vi "LINC Error.vi"(8 "error in (no error)":errorcluster, 10 "expanded error (F)":bool, 11 "LINC session":refnum<class "LINC.lvclass">) -> (0 "error out":errorcluster, 3 "dup LINC session":refnum<class "LINC.lvclass">)   [LabVIEW 2018, in "STEPkgDriver_LINC.lvlib" / "LINC.lvclass"]
uses:
  LINC.lvclass
  STEPkgDriver_LINC.lvlib
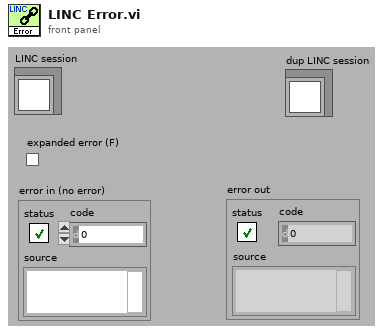
[diagram p1: front panel]
types:
  T1 = cluster{"binary value (F)":bool, "include unit (F)":bool}
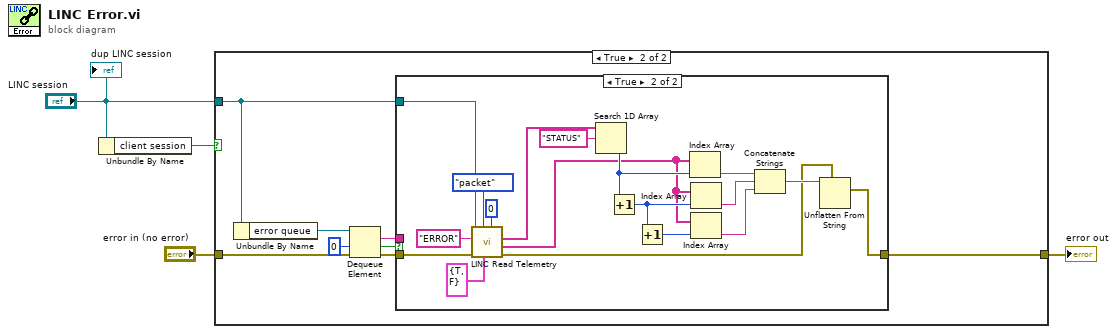
[diagram p0: block diagram]
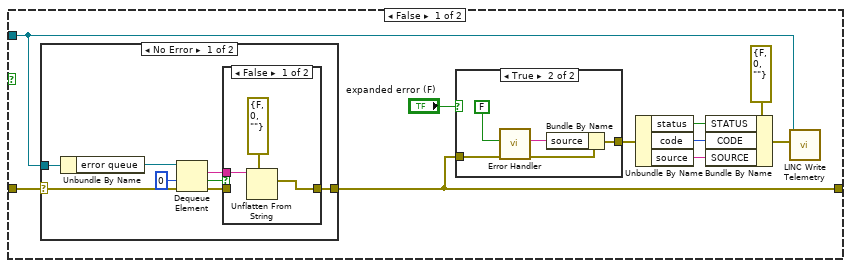
[diagram p2: hidden frame]
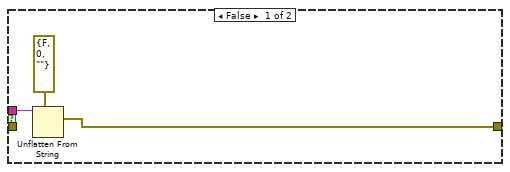
[diagram p6: hidden frame]
diagram:
  n1 = Unbundle By Name("LINC session") -> ("client session"=w3:bool)
  n2 = case shown="True" w3 {
    tunnel: "LINC session" -> [w7 w35]
    tunnel: "error in (no error)" -> [w5 w41]
    tunnel: [w6 w34] -> w1
    frame False {
      n3 = case shown="No Error" w5 {
        selector: w5 -> [w15 w27]
        tunnel: w7 -> [w22 _]
        tunnel: [w17 w27] -> w6
        frame No Error {
          n4 = Unbundle By Name(w22) -> ("error queue"=w21:refnum<queue>)
          n5 = Dequeue Element(queue=w21, timeout in ms (-1)=0, error in (no error)=w15) -> (element=w16:string, timed out?=w18:bool, error out=w19:errorcluster)  [unwired: 1 out]
          n6 = case shown="False" w18 {
            tunnel: w19 -> [_ w26]
            tunnel: [w23 w26] -> w17
            tunnel: w16 -> [w25 _]
            frame False {
              n7 = Unflatten From String(type=errorcluster {"status"=FALSE, "code"=0, "source"=""} ("error out"), binary string=w25) -> (value=w23:errorcluster)  [unwired: 3 in, 2 out]
            }
            frame True {
            }
          }
        }
        frame Error {
        }
      }
      n8 = case shown="True" "expanded error (F)" {
        tunnel: w6 -> [w28 w33]
        tunnel: [w28 w30] -> w9
        frame False {
        }
        frame True {
          n9 = call "Error Handler.vi"("error in (no error)"=w33, "dialog? (T)"=FALSE) -> ("error out"=w31:errorcluster, "error text"=w29:string)  [unwired: 8 in]
          n10 = Bundle By Name(cluster=w31, "source"=w29) -> (w30:errorcluster)
        }
      }
      n11 = Unbundle By Name(w9) -> ("status"=w13:bool, "code"=w12:i32, "source"=w11:string)
      n12 = Bundle By Name(cluster=errorcluster {"STATUS"=FALSE, "CODE"=0, "SOURCE"=""} ("ERROR"), "STATUS"=w13, "CODE"=w12, "SOURCE"=w11) -> (w10:errorcluster)
      n13 = call "LINC Write Telemetry.vi"("packet"=w10, "LINC session"=w7) -> ()  [unwired: 8 in, 2 out]
    }
    frame True {
      n14 = Unbundle By Name(w35) -> ("error queue"=w40:refnum<queue>)
      n15 = Dequeue Element(queue=w40, timeout in ms (-1)=0, error in (no error)=w41) -> (element=w36:string, timed out?=w37:bool, error out=w38:errorcluster)  [unwired: 1 out]
      n16 = case shown="True" w37 {
        tunnel: w38 -> [_ w47]
        tunnel: [w42 w46] -> w34
        tunnel: w36 -> [w44 _]
        tunnel: w35 -> [_ w45]
        frame False {
          n17 = Unflatten From String(type=errorcluster {"status"=FALSE, "code"=0, "source"=""} ("error out"), binary string=w44) -> (value=w42:errorcluster)  [unwired: 3 in, 2 out]
        }
        frame True {
          n18 = call "LINC Read Telemetry.vi"("start field (-1)"=0 ("start field (10)"), "options"=T1 {"binary value (F)"=TRUE, "include unit (F)"=FALSE}, "mode (single)"=enum16{"single", "packet", "all"}."packet", "error in (no error)"=w47, "packet name"="ERROR", "LINC session"=w45) -> ("error out"=w48:errorcluster, "item values"=w53:string[], "item names"=w58:string[])  [unwired: 1 in, 2 out]
          n19 = Search 1D Array(1D array=w58, element="STATUS") -> (index of element=w56:i32)  [unwired: 1 in]
          n20 = Increment(x=w56) -> (x+1=w55:i32)
          n21 = Increment(x=w55) -> (x+1=w54:i32)
          n22 = Index Array(array=w53, index=w56) -> (element=w52:string)
          n23 = Index Array(array=w53, index=w55) -> (element=w51:string)
          n24 = Index Array(array=w53, index=w54) -> (element=w50:string)
          n25 = Concatenate Strings(w52, w51, w50) -> (w49:string)
          n26 = Unflatten From String(type=w48, binary string=w49) -> (value=w46:errorcluster)  [unwired: 3 in, 2 out]
        }
      }
    }
  }
  "error out" <- w1
  "dup LINC session" <- "LINC session"
